vi "hse-application_SystemConfiguration_ValidateFile.vi"(8 "error in (no error)":errorcluster, 11 "Config File":path) -> (0 "error out":errorcluster)   [LabVIEW 2014, in "hse-application.lvclass"]
doc: "Check if <b>Config File</b> exists. If it can't be read, try and copy config.ini.default over to config. ini and show a message. If that also doesn't work, throw an error and show a message."
uses:
  hse-application.lvclass
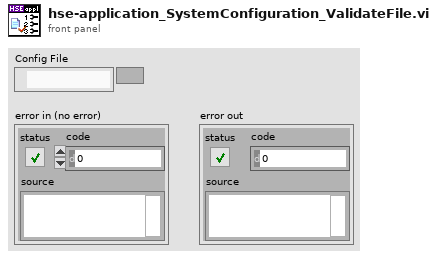
[diagram p1: front panel]
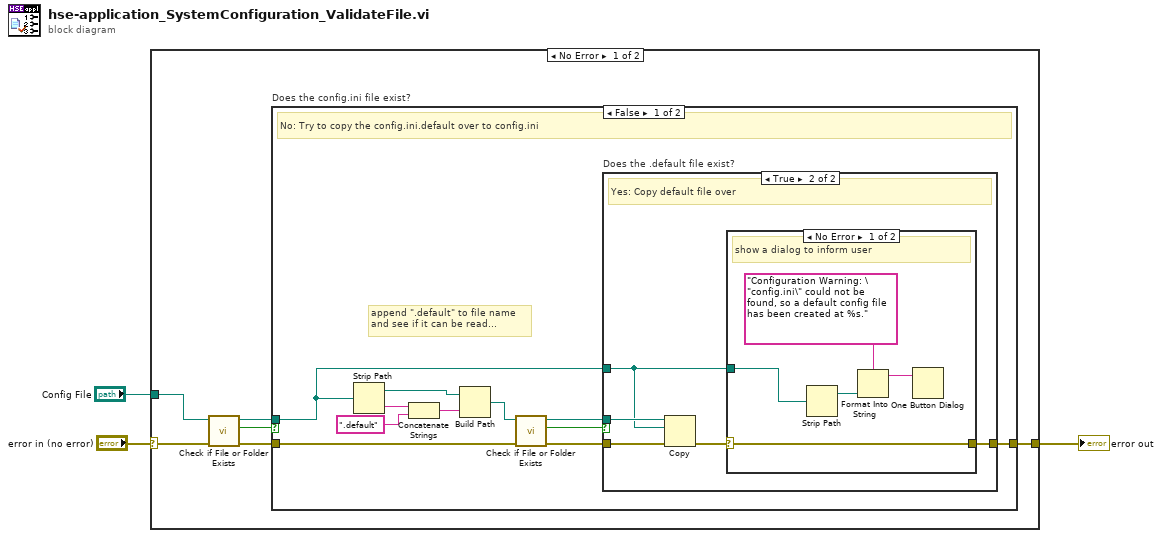
[diagram p0: block diagram]
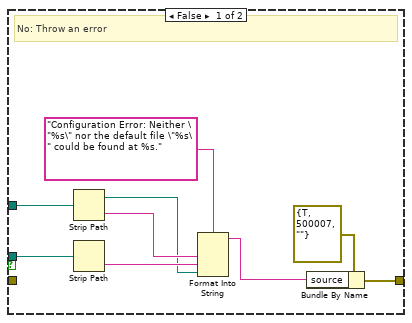
[diagram p2: hidden frame]
diagram:
  n1 = case shown="No Error" "error in (no error)" {
    selector: "error in (no error)" -> [w8 w42]
    tunnel: [w5 w42] -> w2
    tunnel: "Config File" -> [w9 _]
    frame No Error {
      n2 = call <vilib>:"Check if File or Folder Exists.vi"("error in (no error)"=w8, "path"=w9) -> ("error out"=w6:errorcluster, "file or folder exists?"=w7:bool, "dup path"=w4:path)  [unwired: 7 in]
      n3 = case "Does the config.ini file exist?" shown="False" w7 {
        tunnel: w6 -> [w15 w41]
        tunnel: [w10 w41] -> w5
        tunnel: w4 -> [w11 _]
        frame False {
          # "append \".default\" to file name\nand see if it can be read..."
          # "No: Try to copy the config.ini.default over to config.ini"
          n4 = Strip Path(path=w11) -> (stripped path=w19:path, name=w20:string)
          n5 = Concatenate Strings(w20, ".default" ("string")) -> (w18:string)
          n6 = Build Path(base path=w19, name or relative path=w18) -> (appended path=w16:path)
          n7 = call <vilib>:"Check if File or Folder Exists.vi"("error in (no error)"=w15, "path"=w16) -> ("error out"=w14:errorcluster, "file or folder exists?"=w13:bool, "dup path"=w12:path)  [unwired: 7 in]
          n8 = case "Does the .default file exist?" shown="True" w13 {
            tunnel: w14 -> [_ w34]
            tunnel: w12 -> [w24 w33]
            tunnel: w11 -> [w25 w30]
            tunnel: [w28 w31] -> w10
            frame False {
              # "No: Throw an error"
              n9 = Strip Path(path=w25) -> (stripped path=w21:path, name=w22:string)
              n10 = Strip Path(path=w24) -> (name=w23:string)  [unwired: 1 out]
              n11 = Format Into String(format string="Configuration Error: Neither \"%s\" nor the default file \"%s\" could be found at %s.", w22, w23, w21) -> (resulting string=w27:string)  [unwired: 2 in, 1 out]
              n12 = Bundle By Name(cluster=errorcluster {"status"=TRUE, "code"=500007, "source"=""} ("error out"), "source"=w27) -> (w28:errorcluster)
            }
            frame True {
              # "Yes: Copy default file over"
              n13 = Copy(8:w34, 10:w30, 11:w33) -> (0:w32:errorcluster)  [unwired: 2 in, 2 out]
              n14 = case shown="No Error" w32 {
                selector: w32 -> [w39 w40]
                tunnel: [w39 w40] -> w31
                tunnel: w30 -> [w36 _]
                frame No Error {
                  # "show a dialog to inform user"
                  n15 = Strip Path(path=w36) -> (stripped path=w35:path)  [unwired: 1 out]
                  n16 = Format Into String(format string="Configuration Warning: \"config.ini\" could not be found, so a default config file has been created at %s.", w35) -> (resulting string=w37:string)  [unwired: 2 in, 1 out]
                  n17 = One Button Dialog(message=w37) -> ()  [unwired: 1 in, 1 out]
                }
                frame Error {
                }
              }
            }
          }
        }
        frame True {
          # "Yes: Do nothing."
        }
      }
    }
    frame Error {
    }
  }
  "error out" <- w2
